vi "Unit Test.vi"() -> ()   [LabVIEW 2024]
uses:
  <instrlib>/OptoMMP/OptoMMP.lvlib
panel:
  in  "Tab Control":enum32{"Unit Test", "Errors", "Arrays"}(tab)
  out "Test 2":bool
  out "Test 1":bool
  out "Test 3":bool
  out "Test 4":bool
  out "Test 5":bool
  out "Test 6":bool
  out "Test 7":bool
  out "Test 8":bool
  out "Test 9":bool
  out "Test 10":bool
  out "Test 11":bool
  out "Test 12":bool
  out "Test 13":bool
  in  "IP Address":string
  # "Copyright (c) 2025 California Institute of Technology (Caltech).\nU.S. Government sponsorship acknowledged.\n\nLicensed under the Apache License, Version 2.0 (the \"License\");\nyou may not use this file except in compliance with the License.\nYou may obtain a copy of the License at\n\n    http://www.apache.org/licenses/LICENSE-2.0\n\nUnless required by applicable law or agreed to in writing, software\ndistributed under the License is distributed on an \"AS IS\" BASIS,\nWITHOUT WARRANTIES OR CONDITIONS OF ANY KIND, either express or implied.\nSee the License for the specific language governing permissions and\nlimitations under the License."
  # "OptoMMP Driver Unit Testing"
  # "Enter client IP address"
  # "Instructions:\n\n1. Power off Opto 22 controllers. Wait a few seconds, then power back on.\n2. Enter IP address of Opto 22 device.\n3. Run test.\n\nResults: \nAll green indicator lights should be on in systems with analog and digital modules.\n\n4. Run test once more.\n\nResults:\nTest 5, 6, 7, and 8 indicator lights should be off in systems with analog and digital modules"
  # "Space for adding error indicators"
  # "Space for adding data indicators"
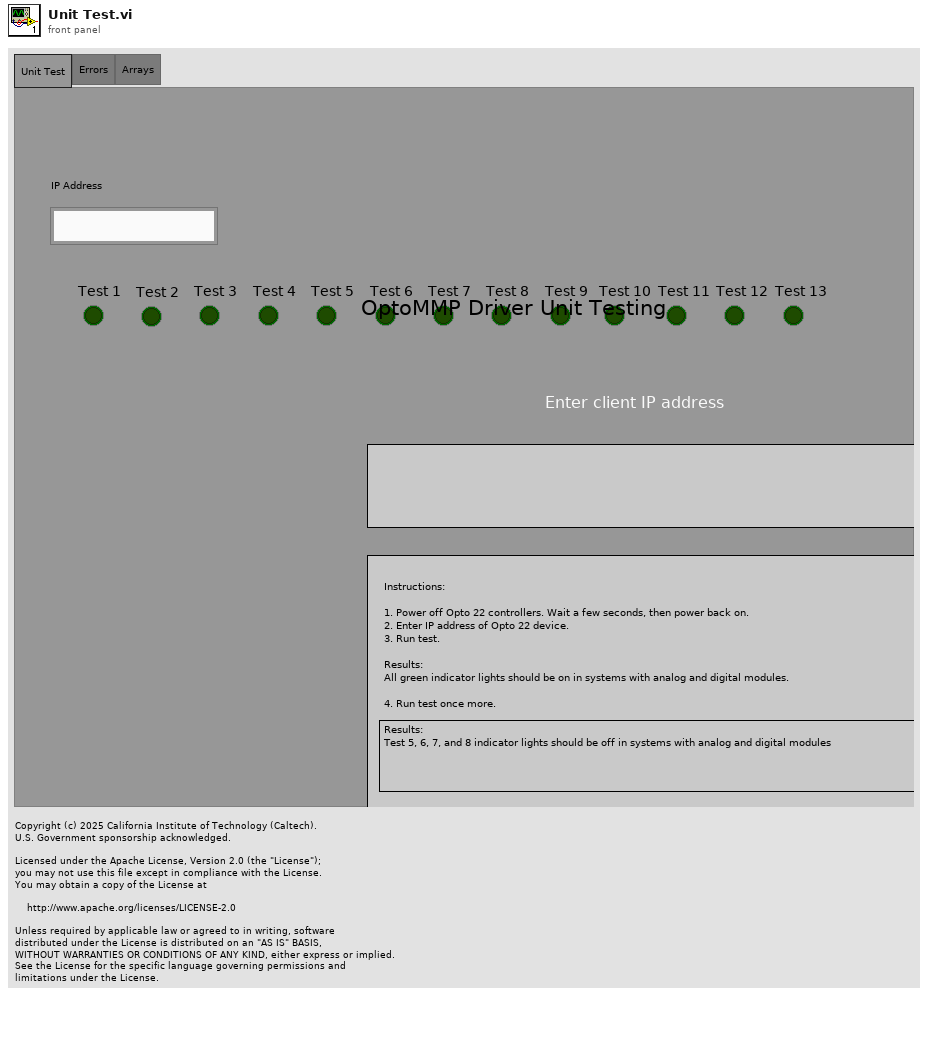
[diagram p1: front panel]
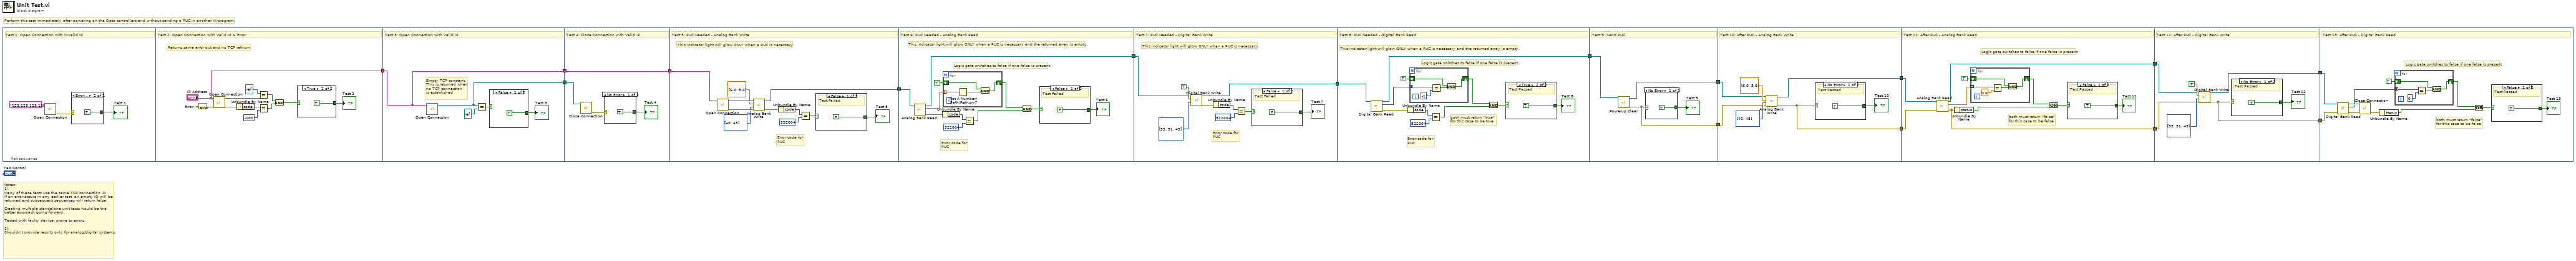
[diagram p0: block diagram]
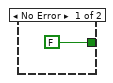
[diagram p2: hidden frame]
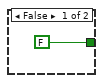
[diagram p3: hidden frame]
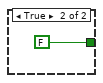
[diagram p4: hidden frame]
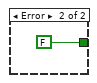
[diagram p5: hidden frame]
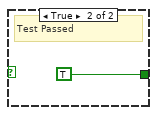
[diagram p6: hidden frame]
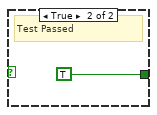
[diagram p7: hidden frame]
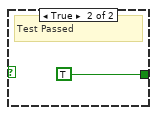
[diagram p8: hidden frame]
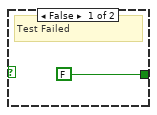
[diagram p9: hidden frame]
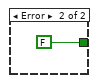
[diagram p10: hidden frame]
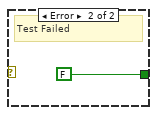
[diagram p11: hidden frame]
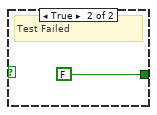
[diagram p12: hidden frame]
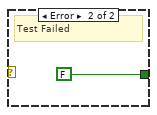
[diagram p13: hidden frame]
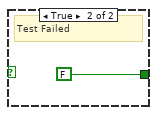
[diagram p14: hidden frame]
diagram:
  # "Notes:\n1).\nMany of these tests use the same TCP connection ID.\nIf an error occurs in any earlier test, an empty ID will be\nreturned and subsequent sequences will return false.\n\nCreating multiple standalone unit tests would be the\nbetter approach going forward. \n\nTested with faulty device; prone to errors.\n\n2). \nShouldn't provide results only for analog/digital systems."
  # "Perform this test immediately after powering on the Opto controllers and without sending a PUC in another VI/program."
  n1 = flat-sequence {
    tunnel: ["IP Address"] -> w3
    tunnel: [w36] -> w16
    tunnel: w3 -> [w35]
    tunnel: [w35] -> w2
    tunnel: w16 -> [w45]
    tunnel: w2 -> [w42]
    tunnel: [w42] -> w1
    tunnel: [w49] -> w15
    tunnel: w1 -> [w48]
    tunnel: w15 -> [w62]
    tunnel: [w61] -> w14
    tunnel: w14 -> [w79]
    tunnel: [w78] -> w13
    tunnel: w13 -> [w92]
    tunnel: [w89] -> w12
    tunnel: w12 -> [w109]
    tunnel: [w108] -> w11
    tunnel: [w107] -> w10
    tunnel: w11 -> [w115]
    tunnel: w10 -> [w116]
    tunnel: [w114] -> w9
    tunnel: [w113] -> w8
    tunnel: w9 -> [w125]
    tunnel: w8 -> [w124]
    tunnel: [w123] -> w7
    tunnel: [w122] -> w6
    tunnel: w7 -> [w141]
    tunnel: w6 -> [w142]
    tunnel: [w140] -> w5
    tunnel: [w139] -> w4
    tunnel: w5 -> [w153]
    tunnel: w4 -> [w152]
    frame #0 {
      # "Test 1: Open Connection with Invalid IP"
      n2 = call <instrlib>:"Open Connection.vi"("Client IP Address"="123.123.123.123") -> ("error out"=w17:errorcluster)  [unwired: 9 in, 1 out]
      n3 = case shown="Error .." w17 {
        tunnel: [FALSE TRUE] -> w19
        frame No Error {
        }
        frame Error {
        }
      }
      "Test 1" <- w19
    }
    frame #1 {
      w31 = errorcluster {"status"=TRUE, "code"=-100, "source"=""}  # Error in
      # "Returns same error out and no TCP refnum"
      # "Test 2: Open Connection with Valid IP & Error"
      n4 = call <instrlib>:"Open Connection.vi"("error in (no error)"=w31, "Client IP Address"="IP Address") -> ("error out"=w23:errorcluster, "TCP Network Connection out"=w24:refnum<k5>)  [unwired: 8 in]
      n5 = Unbundle By Name(w23) -> ("code"=w29:i32)
      n6 = Equal?(x=refnum<k5> refnum ("y"), y=w24) -> (x = y?=w30:bool)
      n7 = Equal?(x=w29, y=-100) -> (x = y?=w27:bool)
      n8 = And(x=w30, y=w27) -> (x .and. y?=w26:bool)
      n9 = case shown="True" w26 {
        tunnel: [FALSE TRUE] -> w32
        frame False {
        }
        frame True {
        }
      }
      "Test 2" <- w32
    }
    frame #2 {
      # "Empty TCP constant.\nThis is returned when\nno TCP connection\nis established"
      # "Test 3: Open Connection with Valid IP"
      n10 = call <instrlib>:"Open Connection.vi"("Client IP Address"=w35) -> ("TCP Network Connection out"=w36:refnum<k5>)  [unwired: 9 in, 1 out]
      n11 = Equal?(x=w36, y=refnum<k5> refnum) -> (x = y?=w38:bool)
      n12 = case shown="False" w38 {
        tunnel: [TRUE FALSE] -> w39
        frame False {
        }
        frame True {
        }
      }
      "Test 3" <- w39
    }
    frame #3 {
      # "Test 4: Close Connection with Valid IP"
      n13 = call <instrlib>:"Close Connection.vi"("TCP Network Connection in"=w45) -> ("error out"=w44:errorcluster)  [unwired: 9 in, 1 out]
      n14 = case shown="No Error" w44 {
        tunnel: [TRUE FALSE] -> w43
        frame No Error {
        }
        frame Error {
        }
      }
      "Test 4" <- w43
    }
    frame #4 {
      # "Error code for\nPUC"
      # "This indicator light will glow ONLY when a PUC is necessary."
      # "Test 5: PUC Needed - Analog Bank Write"
      n15 = call <instrlib>:"Open Connection.vi"("Client IP Address"=w48) -> ("error out"=w54:errorcluster, "TCP Network Connection out"=w55:refnum<k5>)  [unwired: 9 in]
      n16 = call <instrlib>:"Analog Bank Write.vi"("error in (no error)"=w54, "Channels to set"=i32[] [40, 45], "Values to set"=sgl[] [6.0, 5.0], "TCP Network Connection in"=w55) -> ("error out"=w50:errorcluster, "TCP Network Connection out"=w49:refnum<k5>)  [unwired: 6 in]
      n17 = Unbundle By Name(w50) -> ("code"=w51:i32)
      n18 = Equal?(x=w51, y=522004) -> (x = y?=w57:bool)
      n19 = case shown="False" w57 {
        tunnel: [FALSE TRUE] -> w56
        frame False {
          # "Test Failed"
        }
        frame True {
          # "Test Passed"
        }
      }
      "Test 5" <- w56
    }
    frame #5 {
      # "Logic gate switches to false if one false is present"
      # "Error code for\nPUC"
      # "This indicator light will glow ONLY when a PUC is necessary and the returned array is empty."
      # "Test 6: PUC Needed - Analog Bank Read"
      n20 = call <instrlib>:"Analog Bank Read.vi"("TCP Network Connection in"=w62) -> ("error out"=w64:errorcluster, "Measurements"=w65:sgl[], "TCP Network Connection out"=w61:refnum<k5>)  [unwired: 8 in]
      n21 = Unbundle By Name(w64) -> ("code"=w63:i32)
      n22 = for {
        tunnel: w65 -> [w72] mode=indexing
        shift-right: [w75] -> w67
        shift-left: TRUE -> [w74]
        n23 = Not A Number/Path/Refnum?(number/path/refnum=w72) -> (NaN/Path/Refnum?=w73:bool)
        n24 = And(x=w74, y=w73) -> (x .and. y?=w75:bool)
      }
      n25 = Equal?(x=w63, y=522004) -> (x = y?=w69:bool)
      n26 = And(x=w67, y=w69) -> (x .and. y?=w68:bool)
      n27 = case shown="False" w68 {
        tunnel: [FALSE TRUE] -> w70
        frame False {
          # "Test Failed"
        }
        frame True {
          # "Test Passed"
        }
      }
      "Test 6" <- w70
    }
    frame #6 {
      # "This indicator light will glow ONLY when a PUC is necessary."
      # "Error code for\nPUC"
      # "Test 7: PUC Needed - Digital Bank Write"
      n28 = call <instrlib>:"Digital Bank Write.vi"("Channels to set"=i32[] [55, 51, 49], "Value to set"=TRUE, "TCP Network Connection in"=w79) -> ("error out"=w81:errorcluster, "TCP Network Connection out"=w78:refnum<k5>)  [unwired: 7 in]
      n29 = Unbundle By Name(w81) -> ("code"=w80:i32)
      n30 = Equal?(x=w80, y=522004) -> (x = y?=w85:bool)
      n31 = case shown="False" w85 {
        tunnel: [FALSE TRUE] -> w84
        frame False {
          # "Test Failed"
        }
        frame True {
          # "Test Passed"
        }
      }
      "Test 7" <- w84
    }
    frame #7 {
      # "both must return \"true\"\nfor this case to be true"
      # "This indicator light will glow ONLY when a PUC is necessary and the returned array is empty."
      # "Logic gate switches to false if one false is present"
      # "Error code for\nPUC"
      # "Test 8: PUC Needed - Digital Bank Read"
      n32 = call <instrlib>:"Digital Bank Read.vi"("TCP Network Connection in"=w92) -> ("error out"=w90:errorcluster, "States"=w91:i16[], "TCP Network Connection out"=w89:refnum<k5>)  [unwired: 8 in]
      n33 = Unbundle By Name(w90) -> ("code"=w93:i32)
      n34 = for {
        tunnel: w91 -> [w104] mode=indexing
        shift-right: [w103] -> w95
        shift-left: TRUE -> [w101]
        n35 = Equal?(x=w104, y=i16 -1) -> (x = y?=w102:bool)
        n36 = And(x=w101, y=w102) -> (x .and. y?=w103:bool)
      }
      n37 = Equal?(x=w93, y=522004) -> (x = y?=w97:bool)
      n38 = And(x=w95, y=w97) -> (x .and. y?=w96:bool)
      n39 = case shown="True" w96 {
        tunnel: [FALSE TRUE] -> w98
        frame False {
          # "Test Failed"
        }
        frame True {
          # "Test Passed"
        }
      }
      "Test 8" <- w98
    }
    frame #8 {
      # "Test 9: Send PUC"
      n40 = call <instrlib>:"Powerup Clear.vi"("TCP Network Connection in"=w109) -> ("error out"=w107:errorcluster, "connection ID out"=w108:refnum<k5>)  [unwired: 9 in]
      n41 = case shown="No Error" w107 {
        tunnel: [TRUE FALSE] -> w110
        frame No Error {
        }
        frame Error {
        }
      }
      "Test 9" <- w110
    }
    frame #9 {
      # "Test 10: After PUC - Analog Bank Write"
      n42 = call <instrlib>:"Analog Bank Write.vi"("error in (no error)"=w116, "Channels to set"=i32[] [40, 45], "Values to set"=sgl[] [6.0, 5.0], "TCP Network Connection in"=w115) -> ("error out"=w113:errorcluster, "TCP Network Connection out"=w114:refnum<k5>)  [unwired: 6 in]
      n43 = case shown="No Error" w113 {
        tunnel: [TRUE FALSE] -> w119
        frame No Error {
          # "Test Passed"
        }
        frame Error {
          # "Test Failed"
        }
      }
      "Test 10" <- w119
    }
    frame #10 {
      # "both must return \"false\"\nfor this case to be false"
      # "Logic gate switches to false if one false is present"
      # "Test 11: After PUC - Analog Bank Read"
      n44 = call <instrlib>:"Analog Bank Read.vi"("error in (no error)"=w124, "TCP Network Connection in"=w125) -> ("error out"=w122:errorcluster, "Measurements"=w129:sgl[], "TCP Network Connection out"=w123:refnum<k5>)  [unwired: 7 in]
      n45 = Unbundle By Name(w122) -> ("status"=w126:bool)
      n46 = for {
        tunnel: w129 -> [w136] mode=indexing
        shift-right: [w134] -> w128
        shift-left: TRUE -> [w132]
        n47 = Equal?(x=w136, y=sgl 0.0) -> (x = y?=w133:bool)
        n48 = And(x=w132, y=w133) -> (x .and. y?=w134:bool)
      }
      n49 = Or(x=w128, y=w126) -> (x .or. y?=w127:bool)
      n50 = case shown="False" w127 {
        tunnel: [TRUE FALSE] -> w131
        frame False {
          # "Test Passed"
        }
        frame True {
          # "Test Failed"
        }
      }
      "Test 11" <- w131
    }
    frame #11 {
      # "Test 12: After PUC - Digital Bank Write"
      n51 = call <instrlib>:"Digital Bank Write.vi"("error in (no error)"=w142, "Channels to set"=i32[] [55, 51, 49], "Value to set"=TRUE, "TCP Network Connection in"=w141) -> ("error out"=w139:errorcluster, "TCP Network Connection out"=w140:refnum<k5>)  [unwired: 6 in]
      n52 = case shown="No Error" w139 {
        tunnel: [TRUE FALSE] -> w145
        frame No Error {
          # "Test Passed"
        }
        frame Error {
          # "Test Failed"
        }
      }
      "Test 12" <- w145
    }
    frame #12 {
      # "both must return \"false\"\nfor this case to be false"
      # "Logic gate switches to false if one false is present"
      # "Test 13: After PUC - Digital Bank Read"
      n53 = call <instrlib>:"Digital Bank Read.vi"("error in (no error)"=w152, "TCP Network Connection in"=w153) -> ("error out"=w150:errorcluster, "States"=w148:i16[], "TCP Network Connection out"=w151:refnum<k5>)  [unwired: 7 in]
      n54 = call <instrlib>:"Close Connection.vi"("error in (no error)"=w150, "TCP Network Connection in"=w151) -> ("error out"=w149:errorcluster)  [unwired: 8 in, 1 out]
      n55 = Unbundle By Name(w149) -> ("status"=w154:bool)
      n56 = for {
        tunnel: w148 -> [w163] mode=indexing
        shift-right: [w162] -> w156
        shift-left: TRUE -> [w160]
        n57 = Equal?(x=w163, y=i16 0) -> (x = y?=w161:bool)
        n58 = And(x=w160, y=w161) -> (x .and. y?=w162:bool)
      }
      n59 = Or(x=w156, y=w154) -> (x .or. y?=w157:bool)
      n60 = case shown="False" w157 {
        tunnel: [TRUE FALSE] -> w158
        frame False {
          # "Test Passed"
        }
        frame True {
          # "Test Failed"
        }
      }
      "Test 13" <- w158
    }
  }
